vi "Resistance Test_BU.vi"(0 "DMM ref in":refnum<visa-resource-name>, 2 "Resistance Test REF":refnum<vi>, 3 "Resistance Test Stop REF":refnum<vi>, 5 "DMM error in":errorcluster, 7 "Channel  Count":i32, 9 "ESP32 ref in":refnum<visa-resource-name>="COM4", 11 "ESP32 error in":errorcluster, 12 "Wait Current Stable Period":i32, 14 "Current Sense \nResitance Array":dbl[](array[numeric])) -> (1 "Array 2":bool[](array[boolean]), 4 "unsigned 8bit integer":u8, 6 "error?":bool, 8 "Array":dbl[](array[numeric]), 10 "ESP32 ref out":refnum<visa-resource-name>, 15 "ESP32 error out":errorcluster)   [LabVIEW 2023]
uses:
  <instrlib>/Agilent 3446X Series/Agilent 3446X Series.lvlib
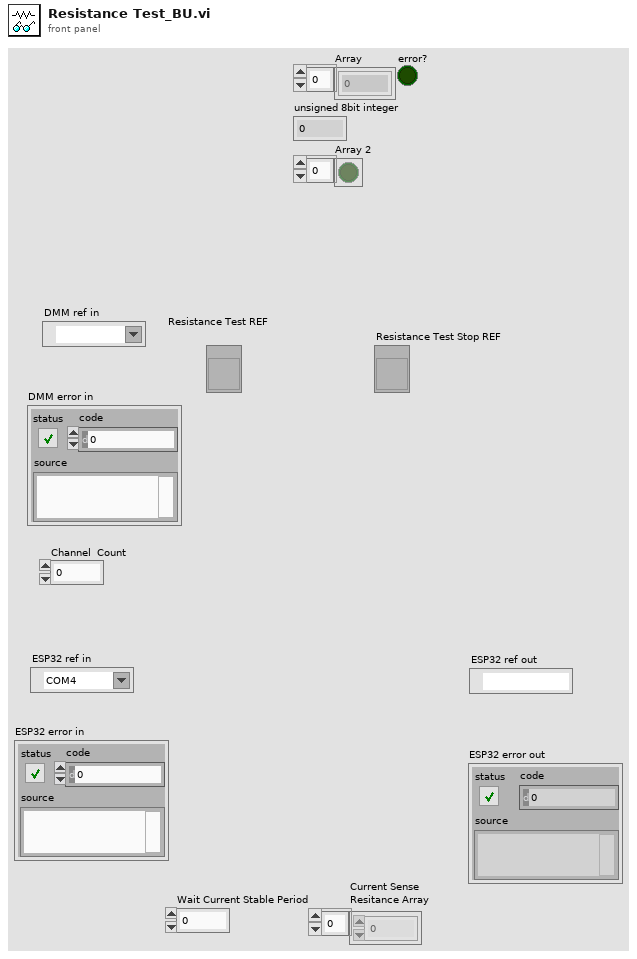
[diagram p1: front panel]
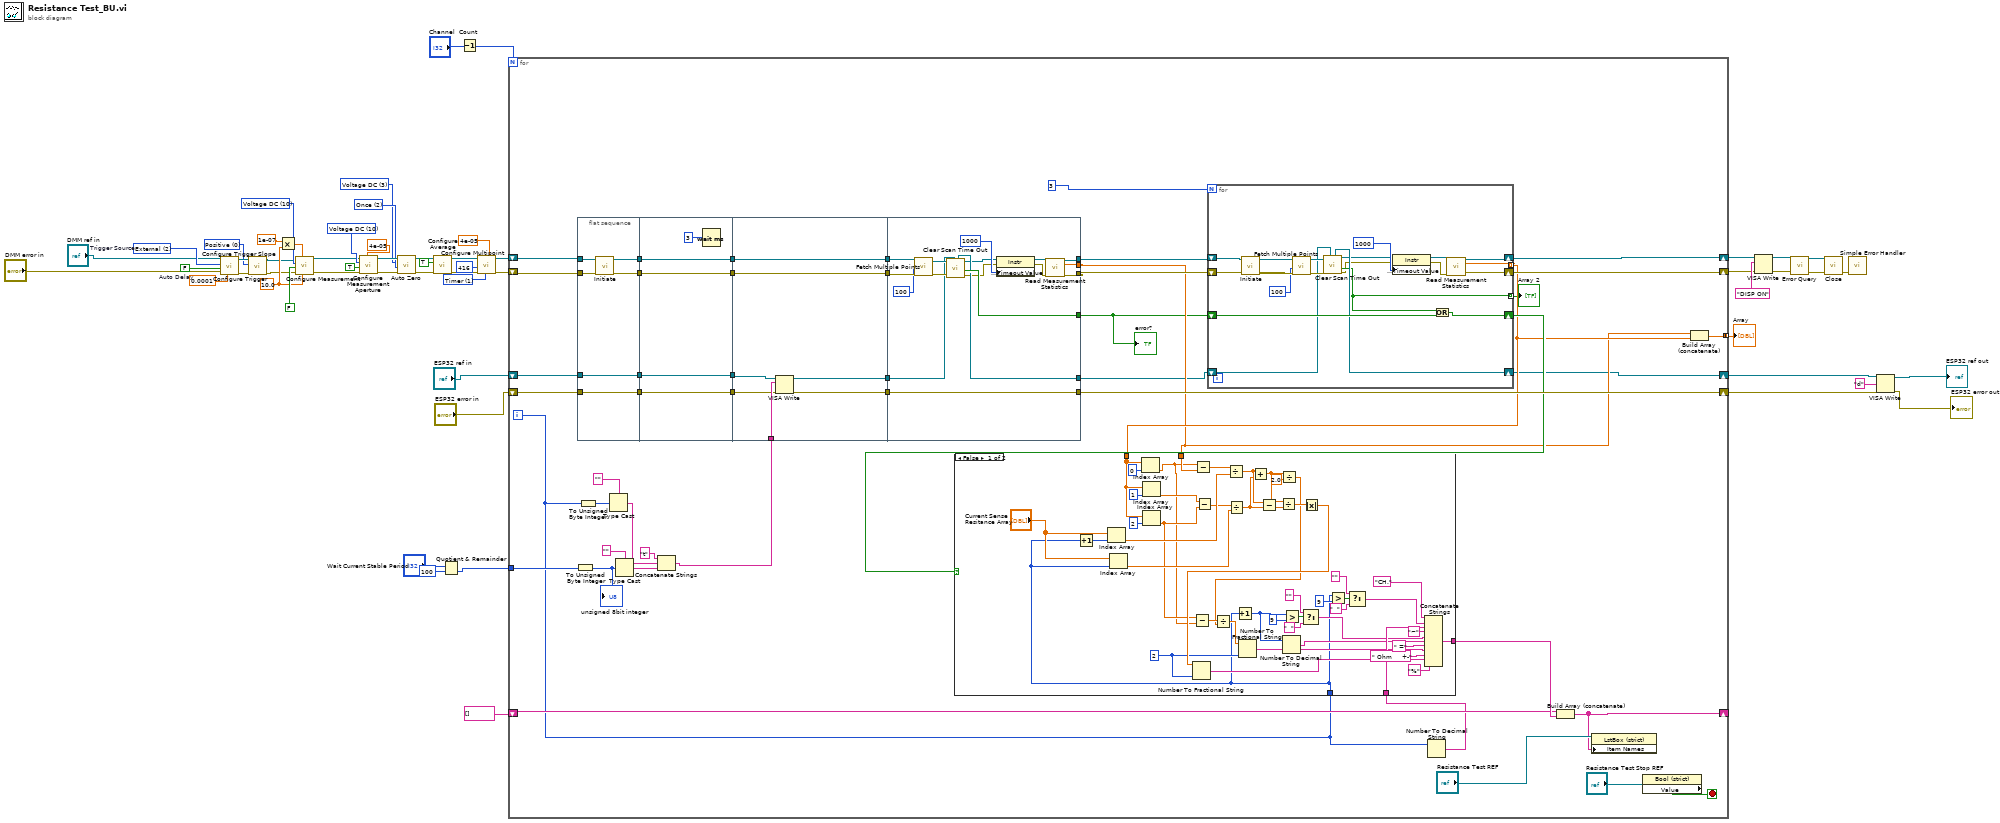
[diagram p0: block diagram]
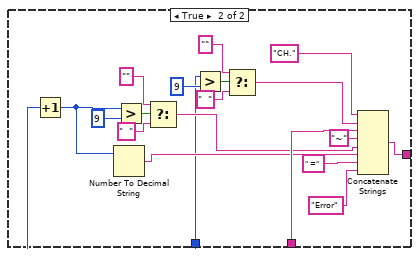
[diagram p2: hidden frame]
diagram:
  w16 = 0 items=["Positive", "Negative"] ("Trigger Edge (1: Negative)")
  w14 = 2 items=["Immediate", "Software (Bus)", "External"]  # Trigger Source
  w15 = FALSE  # Auto Delay
  w19 = 10.0 ("Manual Range (1)")
  w23 = 10 items=["Continuity", "Current AC", "Current DC", "Diode", "Frequency", "Resistance 4-wire", "Period", "Resistance 2-wire", "Temperature", "Voltage AC", "Voltage DC", "Voltage DC Ratio", "Capacitance"] ("Measurement Function (10: Voltage DC)")
  w27 = 1 items=["Immediate", "Timer"] ("Sample Source (0: Immediate)")
  w34 = 3 items=["Current DC", "Resistance", "Temperature", "Voltage DC"] ("Zero Type (0: Current DC)")
  w35 = 2 items=["Disable", "Enable", "Once"] ("Auto Zero (1: Enable)")
  w31 = 10 items=["Continuity", "Current AC", "Current DC", "Diode", "Frequency", "Resistance 4-wire", "Period", "Resistance 2-wire", "Temperature", "Voltage AC", "Voltage DC", "Voltage DC Ratio", "Capacitance"] ("Measurement Function (0: Continuity)")
  n1 = call <instrlib>:"Configure Trigger.vi"("Manual Trigger Delay (1 s)"=0.0001, "error in (no error)"="DMM error in", "Auto Delay (F:Disable)"=w15, "Trigger Source (0: Immediate)"=w14, "VISA resource name"="DMM ref in") -> ("error out"=w18:errorcluster, "VISA resource name out"=w17:refnum<visa-resource-name>)  [unwired: 1 in, 4 out]
  n2 = call <instrlib>:"Configure Trigger Slope.vi"("error in (no error)"=w18, "Trigger Edge (1: Negative)"=w16, "VISA resource name"=w17) -> ("error out"=w11:errorcluster, "VISA resource name out"=w12:refnum<visa-resource-name>)  [unwired: 7 in]
  n3 = Multiply(x=1e-07, y=w19) -> (x*y=w24:dbl)
  n4 = call <instrlib>:"Configure Measurement.vi"("Manual Range (1)"=w19, "Absolute Resolution (1E-6)"=w24, "error in (no error)"=w11, "Auto Range (T: Enable)"=FALSE, "Measurement Function (10: Voltage DC)"=w23, "VISA resource name"=w12) -> ("error out"=w20:errorcluster, "VISA resource name out"=w21:refnum<visa-resource-name>)  [unwired: 4 out]
  n5 = call <instrlib>:"Configure Measurement Aperture.vi"("Aperture Time (0.1s)"=4e-05, "error in (no error)"=w20, "Enable Aperture (F: Disable)"=TRUE, "Measurement Function (0: Continuity)"=w31, "VISA resource name"=w21) -> ("error out"=w38:errorcluster, "VISA resource name out"=w37:refnum<visa-resource-name>)  [unwired: 5 in]
  n6 = call <instrlib>:"Auto Zero.vi"("error in (no error)"=w38, "Auto Zero (1: Enable)"=w35, "Zero Type (0: Current DC)"=w34, "VISA resource name"=w37) -> ("error out"=w40:errorcluster, "VISA resource name out"=w39:refnum<visa-resource-name>)  [unwired: 6 in]
  n7 = call <instrlib>:"Configure Average.vi"("error in (no error)"=w40, "Enable Statistics (F: Disable)"=TRUE, "VISA resource name"=w39) -> ("error out"=w29:errorcluster, "VISA resource name out"=w30:refnum<visa-resource-name>)  [unwired: 7 in]
  n8 = Quotient & Remainder(x="Wait Current Stable Period", y=100) -> (floor(x/y)=w4:i32)  [unwired: 1 out]
  n9 = Decrement(x="Channel  Count") -> (x-1=w2:i32)
  n10 = call <instrlib>:"Configure Multipoint.vi"("Sample Interval (1 Second)"=4e-05, "Sample Source (0: Immediate)"=w27, "error in (no error)"=w29, "Sample Count (1)"=416, "VISA resource name"=w30) -> ("error out"=w9:errorcluster, "VISA resource name out"=w10:refnum<visa-resource-name>)  [unwired: 2 in, 3 out]
  n11 = for {
    N: w2 -> [_]
    shift-right: [w57] -> w42
    shift-left: "ESP32 ref in" -> [w83]
    shift-right: [w67] -> w3
    shift-left: "ESP32 error in" -> [w81]
    shift-right: [w95] -> w43
    shift-left: w9 -> [w87]
    shift-right: [w96] -> w44
    shift-left: w10 -> [w88]
    shift-right: [w98] -> _
    shift-left: string[] [] -> [w100]
    tunnel: w4 -> [w71]
    tunnel: [w61] -> w1 mode=concatenating
    i -> [w65]
    stop <- w102 stop-if-true
    n12 = To Unsigned Byte Integer(number=w71) -> (unsigned 8bit integer=w75:u8)
    "unsigned 8bit integer" <- w75
    n13 = flat-sequence {
      tunnel: w87 -> [w173]
      tunnel: w88 -> [w175]
      tunnel: [w174] -> w94
      tunnel: [w172] -> w93
      tunnel: [w171] -> w84
      tunnel: w83 -> [w171]
      tunnel: w81 -> [w170]
      tunnel: [w170] -> w80
      tunnel: [w180] -> w92
      tunnel: [w179] -> w91
      tunnel: w94 -> [w180]
      tunnel: w93 -> [w179]
      tunnel: w84 -> [w177]
      tunnel: [w177] -> w82
      tunnel: w80 -> [w176]
      tunnel: [w176] -> w79
      tunnel: w92 -> [w187]
      tunnel: [w187] -> w89
      tunnel: w91 -> [w186]
      tunnel: [w186] -> w90
      tunnel: w82 -> [w185]
      tunnel: w79 -> [w183]
      tunnel: w70 -> [w184]
      tunnel: [w182] -> w69
      tunnel: [w181] -> w68
      tunnel: [w201] -> w85
      tunnel: [w202] -> w86
      tunnel: w90 -> [w204]
      tunnel: w89 -> [w203]
      tunnel: [w193] -> w58
      tunnel: w69 -> [w195]
      tunnel: [w199] -> w67
      tunnel: w68 -> [w199]
      tunnel: [w198] -> w62
      tunnel: [w194] -> w59
      frame #0 {
        n14 = call <instrlib>:"Initiate.vi"("error in (no error)"=w173, "VISA resource name"=w175) -> ("error out"=w172:errorcluster, "VISA resource name out"=w174:refnum<visa-resource-name>)  [unwired: 8 out]
      }
      frame #1 {
        n15 = Wait (ms)(milliseconds to wait=u32 3) -> ()  [unwired: 1 out]
      }
      frame #2 {
        n16 = VISA Write(VISA resource name=w185, write buffer=w184, error in (no error)=w183) -> (VISA resource name out=w182:refnum<visa-resource-name>, error out=w181:errorcluster)  [unwired: 1 out]
      }
      frame #3 {
        n17 = call <instrlib>:"Fetch Multiple Points.vi"("error in (no error)"=w204, "Timeout (10000 ms)"=100, "VISA resource name"=w203) -> ("error out"=w196:errorcluster, "VISA resource name out"=w197:refnum<visa-resource-name>)  [unwired: 1 in, 6 out]
        n18 = call "Clear Scan Time Out.vi"("ESP32 ref"=w195, "error in (no error)"=w196, "VISA Refnum in"=w197) -> ("error out"=w190:errorcluster, "error?"=w194:bool, "VISA Refnum out"=w191:refnum<visa-resource-name>, "ESP32 ref out"=w193:refnum<visa-resource-name>)  [unwired: 4 in, 1 out]
        n19 = property class="Instr"(reference=w191, error in=w190, "General Settings:Timeout Value"=u32 1000) -> (reference out=w189:refnum<visa-resource-name>, error out=w188:errorcluster)
        n20 = call <instrlib>:"Read Measurement Statistics.vi"("VISA resource name"=w189, "error in (no error)"=w188) -> ("VISA resource name out"=w202:refnum<visa-resource-name>, "Arithmetic Mean"=w198:dbl, "error out"=w201:errorcluster)  [unwired: 6 in, 5 out]
      }
    }
    n21 = To Unsigned Byte Integer(number=w65) -> (unsigned 8bit integer=w72:u8)
    n22 = Type Cast(type="" ("string"), x=w72) -> (*(type *) &x=w73:string)
    n23 = Type Cast(type="" ("string"), x=w75) -> (*(type *) &x=w74:string)
    n24 = Concatenate Strings("t" ("data in"), w73, w74) -> (w70:string)
    n25 = for {
      N: 3 -> [_]
      tunnel: [w220] -> w63 mode=indexing
      shift-right: [w218] -> w96
      shift-left: w86 -> [w222]
      shift-right: [w217] -> w95
      shift-left: w85 -> [w221]
      shift-right: [w215] -> w64
      shift-left: w59 -> [w216]
      tunnel: [w210] -> w60 mode=indexing
      shift-right: [w211] -> w57
      shift-left: w58 -> [w212]
      n26 = call <instrlib>:"Initiate.vi"("error in (no error)"=w221, "VISA resource name"=w222) -> ("error out"=w224:errorcluster, "VISA resource name out"=w223:refnum<visa-resource-name>)  [unwired: 8 out]
      n27 = call <instrlib>:"Fetch Multiple Points.vi"("error in (no error)"=w224, "Timeout (10000 ms)"=100, "VISA resource name"=w223) -> ("error out"=w213:errorcluster, "VISA resource name out"=w214:refnum<visa-resource-name>)  [unwired: 1 in, 6 out]
      n28 = call "Clear Scan Time Out.vi"("ESP32 ref"=w212, "error in (no error)"=w213, "VISA Refnum in"=w214) -> ("error out"=w205:errorcluster, "error?"=w210:bool, "VISA Refnum out"=w206:refnum<visa-resource-name>, "ESP32 ref out"=w211:refnum<visa-resource-name>)  [unwired: 4 in, 1 out]
      n29 = property class="Instr"(reference=w206, error in=w205, "General Settings:Timeout Value"=u32 1000) -> (reference out=w208:refnum<visa-resource-name>, error out=w207:errorcluster)
      n30 = Or(x=w210, y=w216) -> (x .or. y?=w215:bool)
      n31 = call <instrlib>:"Read Measurement Statistics.vi"("VISA resource name"=w208, "error in (no error)"=w207) -> ("VISA resource name out"=w218:refnum<visa-resource-name>, "Arithmetic Mean"=w220:dbl, "error out"=w217:errorcluster)  [unwired: 6 in, 5 out]
    }
    "Array 2" <- w60
    n32 = Number To Decimal String(number=w65) -> (decimal integer string=w66:string)  [unwired: 1 in]
    n33 = case shown="False" w64 {
      tunnel: [w145 w164] -> w101
      tunnel: w66 -> [w142 w161]
      tunnel: w63 -> [w130 _]
      tunnel: w65 -> [w104 w152]
      tunnel: w62 -> [w123 _]
      frame False {
        w112 = i16 2 ("precision (6)")
        n34 = Increment(x=w104) -> (x+1=w126:i32)
        n35 = Index Array(array="Current Sense \nResitance Array", index=w126) -> (element=w124:dbl)
        n36 = Index Array(array="Current Sense \nResitance Array", index=w104) -> (element=w121:dbl)
        n37 = Index Array(array=w130, index=0) -> (element=w108:dbl)
        n38 = Index Array(array=w130, index=1) -> (element=w109:dbl)
        n39 = Index Array(array=w130, index=2) -> (element=w110:dbl)
        n40 = Subtract(x=w110, y=w108) -> (x-y=w107:dbl)
        n41 = Subtract(x=w108, y=w123) -> (x-y=w127:dbl)
        n42 = Subtract(x=w109, y=w110) -> (x-y=w122:dbl)
        n43 = Divide(x=w127, y=w124) -> (x/y=w119:dbl)
        n44 = Divide(x=w122, y=w121) -> (x/y=w118:dbl)
        n45 = Increment(x=w104) -> (x+1=w135:i32)
        n46 = Add(x=w119, y=w118) -> (x+y=w116:dbl)
        n47 = Subtract(x=w119, y=w118) -> (x-y=w117:dbl)
        n48 = Divide(x=w116, y=w117) -> (x/y=w115:dbl)
        n49 = Divide(x=w116, y=2.0) -> (x/y=w106:dbl)
        n50 = Divide(x=w107, y=w106) -> (x/y=w105:dbl)
        n51 = Number To Fractional String(number=w105, precision (6)=w112) -> (F-format string=w114:string)  [unwired: 2 in]
        n52 = Number To Decimal String(number=w135) -> (decimal integer string=w134:string)  [unwired: 1 in]
        n53 = Greater?(x=w135, y=9) -> (0:w139:bool)
        n54 = Select(t="" ("string"), s=w139, f="  " ("string")) -> (s? t:f=w136:string)
        n55 = Absolute Value(x=w115) -> (abs(x)=w113:dbl)
        n56 = Number To Fractional String(number=w113, precision (6)=w112) -> (F-format string=w111:string)  [unwired: 2 in]
        n57 = Greater?(x=w104, y=9) -> (0:w148:bool)
        n58 = Select(t="" ("string"), s=w148, f="  " ("string")) -> (s? t:f=w143:string)
        n59 = Concatenate Strings("CH." ("string"), w143, w142, "~" ("string"), w136, w134, " =" ("string"), w114, " Ohm     +-" ("string"), w111, "%" ("string")) -> (w145:string)
      }
      frame True {
        n60 = Increment(x=w152) -> (x+1=w154:i32)
        n61 = Number To Decimal String(number=w154) -> (decimal integer string=w153:string)  [unwired: 1 in]
        n62 = Greater?(x=w154, y=9) -> (0:w158:bool)
        n63 = Select(t="" ("string"), s=w158, f="  " ("string")) -> (s? t:f=w155:string)
        n64 = Greater?(x=w152, y=9) -> (0:w167:bool)
        n65 = Select(t="" ("string"), s=w167, f="  " ("string")) -> (s? t:f=w162:string)
        n66 = Concatenate Strings("CH." ("string"), w162, w161, "~" ("string"), w155, w153, " =" ("string"), "Error" ("string")) -> (w164:string)
      }
    }
    n67 = Build Array (concatenate)(w100, w101) -> (w98:string[])
    n68 = property class="LstBox (strict)"(reference="Resistance Test REF", "Item Names"=w98) -> ()  [unwired: 1 in, 2 out]
    n69 = property class="Bool (strict)"(reference="Resistance Test Stop REF") -> ("Value"=w102:bool)  [unwired: 1 in, 2 out]
    n70 = Build Array (concatenate)(w62, w63) -> (w61:dbl[])
    "error?" <- w59
  }
  "Array" <- w1
  n71 = VISA Write(VISA resource name=w44, write buffer="DISP ON", error in (no error)=w43) -> (VISA resource name out=w51:refnum<visa-resource-name>, error out=w50:errorcluster)  [unwired: 1 out]
  n72 = call <instrlib>:"Error Query.vi"("error in (no error)"=w50, "VISA resource name"=w51) -> ("error out"=w56:errorcluster, "VISA resource name out"=w55:refnum<visa-resource-name>)  [unwired: 8 out]
  n73 = call <instrlib>:"Close.vi"("error in (no error)"=w56, "VISA resource name"=w55) -> ("error out"=w54:errorcluster)  [unwired: 9 out]
  n74 = call <vilib>:"Simple Error Handler.vi"("error in (no error)"=w54) -> ()  [unwired: 1 in, 8 out]
  n75 = VISA Write(VISA resource name=w42, write buffer="d" ("data in"), error in (no error)=w3) -> (VISA resource name out=→"ESP32 ref out":refnum<visa-resource-name>, error out=→"ESP32 error out":errorcluster)  [unwired: 1 out]
